vi "SRV_Wait for Zero IMJ Requests.vi"(0 "Number of IMJ Requests ref":refnum<vi>, 1 "#IMJ semaphore ref":T1, 9 "Timeout (2 s)":dbl=2.0, 11 "error in (no error)":errorcluster, 12 "Reset Count on Timeout? (T)":bool=TRUE) -> (3 "#IMJ semaphore ref out":T1, 4 "Number of IMJ Requests ref out":refnum<vi>, 15 "error out":errorcluster)   [LabVIEW 2009]
doc: "Waits for the Number of IMJ Requests to equal zero.\n\n\nAuthor: Mike Schultz - Logic PD"
uses:
  SRV_Number of IMJ Requests Methods.ctl
panel:
  out "Timed Out?":bool
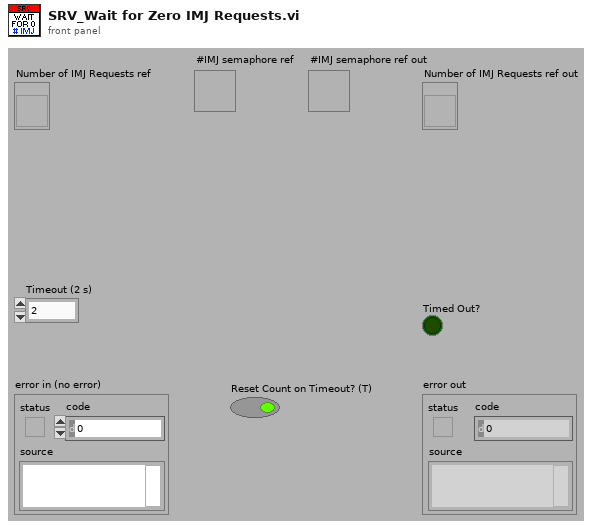
[diagram p1: front panel]
types:
  T1 = typedef "Semaphore RefNum" = refnum<k1>
  T2 = typedef "SRV_Number of IMJ Requests Methods.ctl" = enum16{"Read", "Increment", "Decrement", "Reset", "Close"}
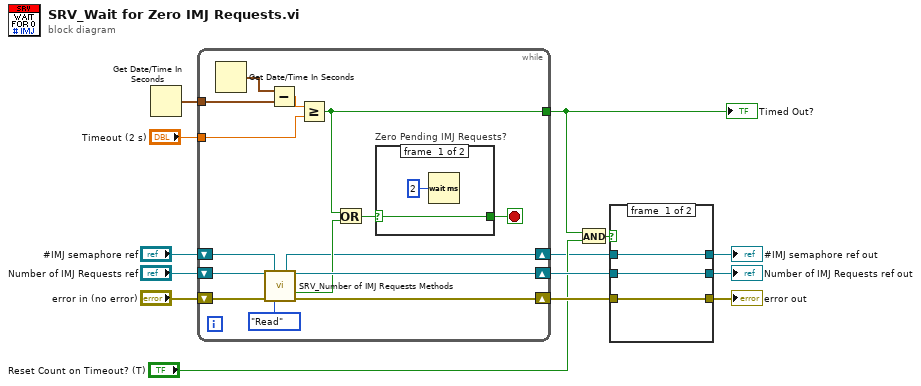
[diagram p0: block diagram]
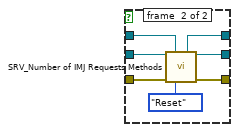
[diagram p2: hidden frame]
diagram:
  n1 = Get Date/Time In Seconds() -> (seconds since 1Jan1904=w12:timestamp)
  n2 = while {
    shift-right: [w27] -> w10
    shift-left: "error in (no error)" -> [w28]
    shift-right: [w25] -> w8
    shift-left: "Number of IMJ Requests ref" -> [w26]
    tunnel: w12 -> [w22]
    tunnel: "Timeout (2 s)" -> [w20]
    tunnel: [w17] -> w6
    shift-right: [w15] -> w2
    shift-left: "#IMJ semaphore ref" -> [w16]
    stop <- w29 stop-if-true
    n3 = Get Date/Time In Seconds() -> (seconds since 1Jan1904=w23:timestamp)
    n4 = call "SRV_Number of IMJ Requests Methods.vi"("Number of IMJ Requests ref"=w26, "semaphore ref"=w16, "error in (no error)"=w28, "Number of IMJ Requests Methods (Read)"=SRV_Number_of_IMJ_Requests_Methods."Read") -> ("semaphore ref out"=w15:T1, "Number of IMJ Requests ref out"=w25:refnum<vi>, "Zero Requests?"=w19:bool, "error out"=w27:errorcluster)  [unwired: 7 in, 1 out]
    n5 = Subtract(x=w23, y=w22) -> (x-y=w21:dbl)
    n6 = Greater Or Equal?(x=w21, y=w20) -> (x >= y?=w17:bool)
    n7 = Or(x=w17, y=w19) -> (x .or. y?=w18:bool)
    n8 = case "Zero Pending IMJ Requests?" shown="False" w18 {
      selector: w18 -> [w31 w32]
      tunnel: [w31 w32] -> w29
      frame #0 {
        n9 = Wait (ms)(milliseconds to wait=u32 2) -> ()  [unwired: 1 out]
      }
      frame #1 {
      }
    }
  }
  "Timed Out?" <- w6
  n10 = And(x=w6, y="Reset Count on Timeout? (T)") -> (x .and. y?=w5:bool)
  n11 = case shown="True" w5 {
    tunnel: w10 -> [w35 w41]
    tunnel: [w35 w40] -> w9
    tunnel: w8 -> [w34 w39]
    tunnel: [w34 w38] -> w7
    tunnel: w2 -> [w33 w37]
    tunnel: [w33 w36] -> w1
    frame #0 {
    }
    frame #1 {
      n12 = call "SRV_Number of IMJ Requests Methods.vi"("Number of IMJ Requests ref"=w39, "semaphore ref"=w37, "error in (no error)"=w41, "Number of IMJ Requests Methods (Read)"=SRV_Number_of_IMJ_Requests_Methods."Reset") -> ("semaphore ref out"=w36:T1, "Number of IMJ Requests ref out"=w38:refnum<vi>, "error out"=w40:errorcluster)  [unwired: 7 in, 2 out]
    }
  }
  "error out" <- w9
  "Number of IMJ Requests ref out" <- w7
  "#IMJ semaphore ref out" <- w1
